vi "IntegraMeter_ReadEnergy.vi"(8 "error in (no error)":errorcluster, 11 "VISA resource name":refnum<visa-resource-name>) -> (0 "error out":errorcluster, 2 "Laser Energy (J)":dbl, 3 "VISA resource name out":refnum<visa-resource-name>)   [LabVIEW 2024]
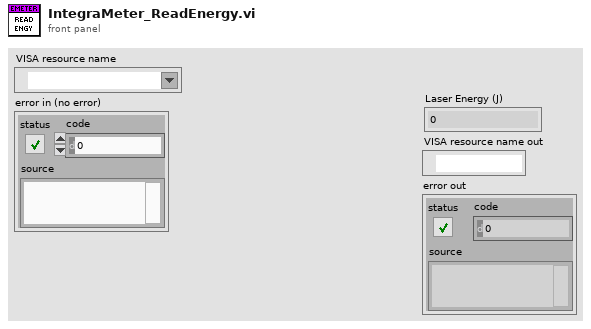
[diagram p1: front panel]
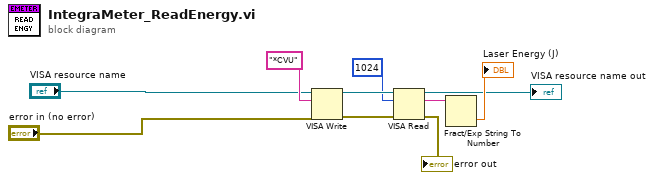
[diagram p0: block diagram]
diagram:
  n1 = VISA Write(VISA resource name="VISA resource name", write buffer="*CVU", error in (no error)="error in (no error)") -> (VISA resource name out=w10:refnum<visa-resource-name>, error out=w1:errorcluster)  [unwired: 1 out]
  n2 = VISA Read(VISA resource name=w10, byte count=u32 1024, error in (no error)=w1) -> (VISA resource name out=→"VISA resource name out":refnum<visa-resource-name>, read buffer=w7:string, error out=→"error out":errorcluster)  [unwired: 1 out]
  n3 = Fract/Exp String To Number(string=w7) -> (number=→"Laser Energy (J)":dbl)  [unwired: 3 in, 1 out]
